vi "Configure Fans.vi"(8 "error in":errorcluster, 11 "tCRD in":refnum<class "Open Path CRD.lvclass">) -> (0 "error out":errorcluster, 3 "tCRD out":refnum<class "Open Path CRD.lvclass">)   [LabVIEW 2015, in "Open Path CRD.lvclass"]
uses:
  Open Path CRD.lvclass
  Reusable/Session APIs/File Access/Config Data/Config Data.lvclass
  Reusable/Instrument/Instrument.lvclass/Instrument.ctl
  Reusable/Session APIs/File Access/Config Data/Config Data.lvclass/Config Data.ctl
  Reusable/Instrument/Read Cfg Session.vi
  Reusable/Session APIs/File Access/Config Data/Accessors/Read Ref.vi
  <vilib>/Utility/config.llb/Read Key (Boolean).vi
  <vilib>/Utility/config.llb/Read Key (Double).vi
  <userlib>/_Session Fwk/Session - Root.lvclass
  <vilib>/Utility/config.llb/NI_LVConfig.lvlib
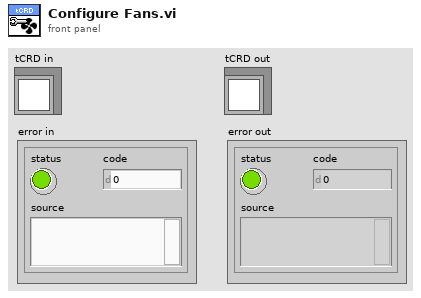
[diagram p1: front panel]
types:
  T1 = typedef "Session - Root.lvclass/Session Handle.ctl" = refnum<data-value>
  T2 = typedef "NI_LVConfig.lvlib/Config Data RefNum.ctl" = refnum<k1>
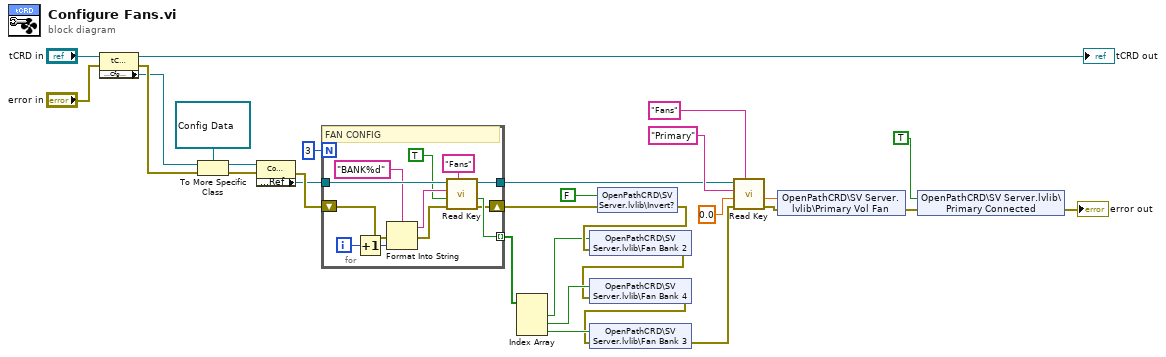
[diagram p0: block diagram]
diagram:
  n1 = property class="tCRD"(reference="tCRD in", error in="error in") -> (reference out=→"tCRD out":refnum<class "Open Path CRD.lvclass">, error out=w27:errorcluster, "Accessors:Cfg Session"=w24:T1)
  n2 = To More Specific Class(target class=refnum<data-value> refnum, reference=w24, error in=w27) -> (specific class reference=w26:refnum<data-value>, error out=w28:errorcluster)
  n3 = property class="Config Data"(reference=w26, error in=w28) -> (error out=w13:errorcluster, "Accessors:Ref"=w12:T2)  [unwired: 1 out]
  n4 = for {
    N: 3 -> [_]
    tunnel: w12 -> [w42]
    tunnel: [w36] -> w11 mode=indexing
    tunnel: [w34] -> w16
    shift-right: [w32] -> w15
    shift-left: w13 -> [w31]
    i -> [w40]
    # "FAN CONFIG"
    n5 = Increment(x=w40) -> (x+1=w39:i32)
    n6 = Format Into String(format string="BANK%d", error in=w31, w39) -> (resulting string=w37:string, error out=w33:errorcluster)  [unwired: 1 in]
    n7 = call-poly <vilib>:"Read Key.vi"("section"="Fans", "error in (no error)"=w33, "default value"=TRUE, "key"=w37, "refnum"=w42) -> ("error out"=w32:errorcluster, "value"=w36:bool, "refnum out"=w34:T2)  [unwired: 3 in, 1 out]
  }
  n8 = Index Array(array=w11) -> (element #1=w6:bool, element #2=w7:bool, element #3=w8:bool)  [unwired: 3 in]
  n9 = shared-variable "OpenPathCRD\\SV Server.lvlib\\Invert?"(FALSE ("Invert?"), error in=w15) -> (error out=w14:errorcluster)
  n10 = shared-variable "OpenPathCRD\\SV Server.lvlib\\Fan Bank 2"(w6, error in=w14) -> (error out=w4:errorcluster)
  n11 = shared-variable "OpenPathCRD\\SV Server.lvlib\\Fan Bank 4"(w7, error in=w4) -> (error out=w5:errorcluster)
  n12 = shared-variable "OpenPathCRD\\SV Server.lvlib\\Fan Bank 3"(w8, error in=w5) -> (error out=w19:errorcluster)
  n13 = call-poly <vilib>:"Read Key.vi"("section"="Fans", "error in (no error)"=w19, "default value"=0.0, "key"="Primary", "refnum"=w16) -> ("error out"=w21:errorcluster, "value"=w30:dbl)  [unwired: 3 in, 2 out]
  n14 = shared-variable "OpenPathCRD\\SV Server.lvlib\\Primary Vol Fan"(w30, error in=w21) -> (error out=w2:errorcluster)
  n15 = shared-variable "OpenPathCRD\\SV Server.lvlib\\Primary Connected"(TRUE ("Primary Connected"), error in=w2) -> (error out=→"error out":errorcluster)
